vi "LSI336Data_terminate.vi"(8 "error in (no error)":errorcluster, 11 "LSI336Data in":refnum<class "LSI336Data.lvclass">) -> (0 "error out":errorcluster, 3 "LSI336Data out":refnum<class "LSI336Data.lvclass">)   [LabVIEW 2020, in "LSI336Data.lvclass"]
uses:
  LSI336Data.lvclass
  LSI336Data.lvclass/LSI336Data.ctl
  istr.lib/Lake Shore 336/Lake Shore 336.lvlib
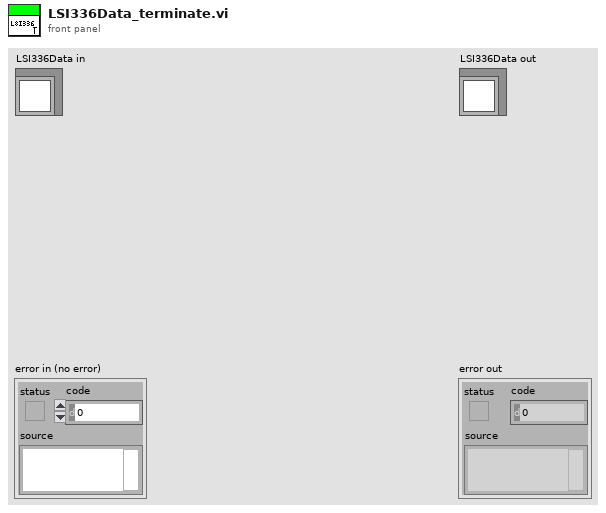
[diagram p1: front panel]
types:
  T1 = enum16{"Initialized", "Ready", "Measuring", "Terminated"}
  T2 = cluster{"LSIName":string, "Labels":string[], "SensorLocations":enum16{"N.C.", "T3He1-1", "T3He1-2", "T3He1-3", "T3He1-4", "T3He2-1", "T3He2-2", "T3He3", "T3He4", "T3He5", "T3He6-1", "T3He6-2", "T3He7-1", "T3He7-2", "T3He8", "T3He9", "T3He10", "T4He1", "T4He2-1", "T4He2-2", "T4He3-1", "T4He3-2", "T4He3-3", "T4He3-4", "T4He4", "T4He5", "T4He6", "T4He7", "T4He8", "T4He9", "T4He10", "T1K1", "T1K2", "T1K3-1", "T1K3-2", "T1K4", "T1K5", "T1K6", "TIP1", "TIP2", "TIP3", "TIP4", "TIP5", "TIP6", "TIP7", "TTH1", "TTH2", "TTH3", "TTH4"}[], "Active?":bool, "VISA res. name":refnum<visa-resource-name>}[]
  T3 = cluster{"LSIName":string, "Labels":string[], "SensorLocations":enum16{"N.C.", "T3He1-1", "T3He1-2", "T3He1-3", "T3He1-4", "T3He2-1", "T3He2-2", "T3He3", "T3He4", "T3He5", "T3He6-1", "T3He6-2", "T3He7-1", "T3He7-2", "T3He8", "T3He9", "T3He10", "T4He1", "T4He2-1", "T4He2-2", "T4He3-1", "T4He3-2", "T4He3-3", "T4He3-4", "T4He4", "T4He5", "T4He6", "T4He7", "T4He8", "T4He9", "T4He10", "T1K1", "T1K2", "T1K3-1", "T1K3-2", "T1K4", "T1K5", "T1K6", "TIP1", "TIP2", "TIP3", "TIP4", "TIP5", "TIP6", "TIP7", "TTH1", "TTH2", "TTH3", "TTH4"}[], "Active?":bool, "VISA res. name":refnum<visa-resource-name>}
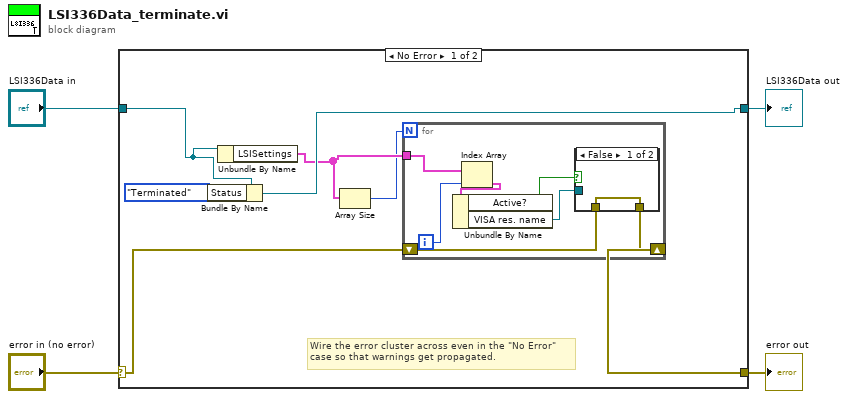
[diagram p0: block diagram]
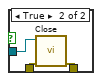
[diagram p2: hidden frame]
diagram:
  n1 = case shown="No Error" "error in (no error)" {
    selector: "error in (no error)" -> [w8 w24]
    tunnel: [w7 w24] -> w3
    tunnel: [w9 w23] -> w1
    tunnel: "LSI336Data in" -> [w11 w23]
    frame No Error {
      # "Wire the error cluster across even in the \"No Error\"\ncase so that warnings get propagated."
      n2 = Bundle By Name(cluster=w11, "Status"=T1."Terminated") -> (w9:refnum<class "LSI336Data.lvclass">)
      n3 = Unbundle By Name(w11) -> ("LSISettings"=w6:T2)
      n4 = Array Size(array=w6) -> (size(s)=w5:i32)
      n5 = for {
        N: w5 -> [_]
        tunnel: w6 -> [w18]
        shift-right: [w12] -> w7
        shift-left: w8 -> [w13]
        i -> [w17]
        n6 = Index Array(array=w18, index=w17) -> (element=w16:T3)
        n7 = Unbundle By Name(w16) -> ("Active?"=w15:bool, "VISA res. name"=w14:refnum<visa-resource-name>)
        n8 = case shown="False" w15 {
          tunnel: w14 -> [_ w22]
          tunnel: w13 -> [w19 w21]
          tunnel: [w19 w20] -> w12
          frame False {
          }
          frame True {
            n9 = call "Close.vi"("error in (no error)"=w21, "VISA resource name"=w22) -> ("error out"=w20:errorcluster)  [unwired: 9 in]
          }
        }
      }
    }
    frame Error {
    }
  }
  "error out" <- w3
  "LSI336Data out" <- w1
